vi "ReadSamples.vi"(8 "error in (no error)":errorcluster, 9 "Max num samples to keep":u32, 10 "Num samples to read":u32, 11 "FpgaRef5782 in":refnum<class "FpgaRef5782.lvclass">) -> (0 "error out":errorcluster, 2 "Data":dbl[][](array[numeric]), 3 "FpgaRef5782 out":refnum<class "FpgaRef5782.lvclass">)   [LabVIEW 2018, in "FpgaRef5782.lvclass"]
uses:
  FpgaRef5782.lvclass
  FpgaRef5782.lvclass/FpgaRef5782.ctl
  <vilib>/Utility/error.llb/Error Cluster From Error Code.vi
  <vilib>/rvi/errors/niLvFpgaAdjustHostInterfaceError.vi
  <vilib>/rvi/interface/nirviMethod/nirviMethod.xnode
  5782 FPGA ref.ctl
  <vilib>/FPGAPlugInAG/Dynamic/niLvFpga_ReadFifo_Dynamic.vi
  <vilib>/rvi/errors/niLvFpgaMergeErrorWithErrorCode.vi
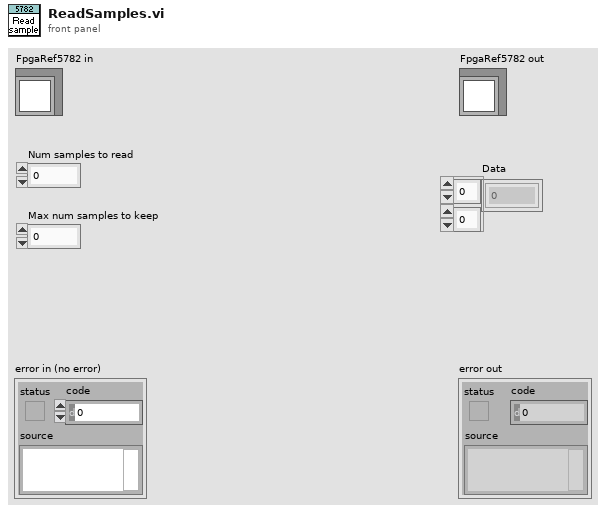
[diagram p1: front panel]
types:
  T1 = typedef "5782 FPGA ref.ctl" = refnum<k20>
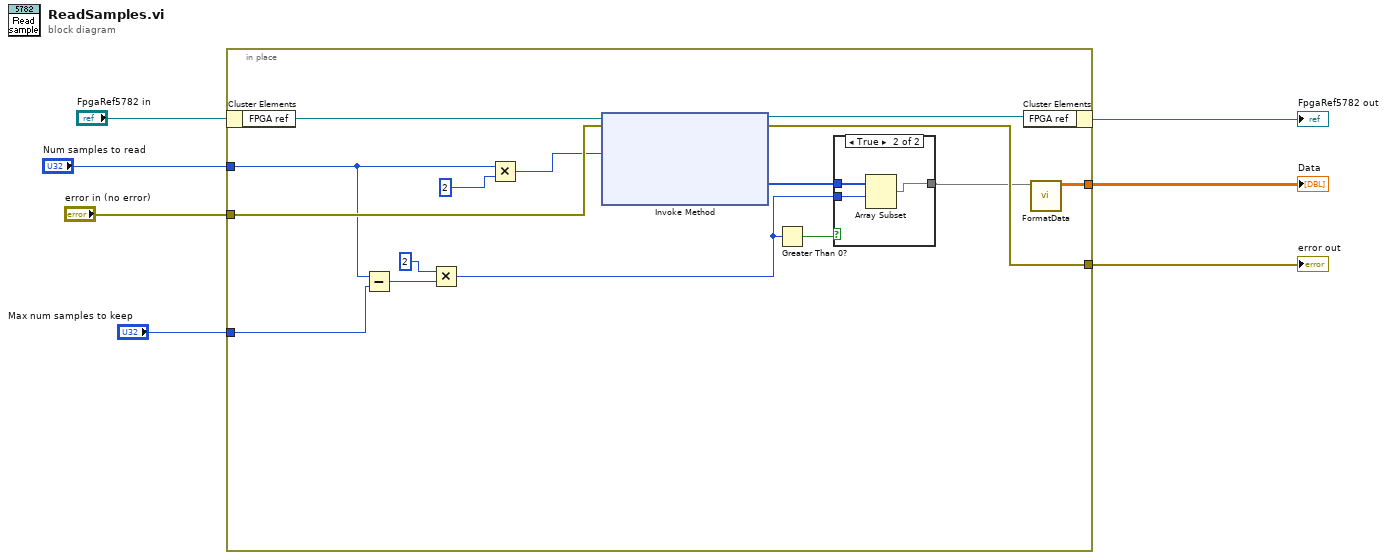
[diagram p0: block diagram]
diagram:
  n1 = in-place {
    in-place-border: [w21] -> w5
    in-place-border: [w20] -> w2
    in-place-border: "Num samples to read" -> [w9]
    in-place-border: "error in (no error)" -> [w18]
    in-place-border: "Max num samples to keep" -> [w10]
    n2 = in-place-cluster #1("FpgaRef5782 in") -> ("FPGA ref"=w19:T1)
    n3 = Subtract(x=w9, y=w10) -> (x-y=w15:u32)
    n4 = Multiply(x=u32 2, y=w15) -> (x*y=w14:u32)
    n5 = Multiply(x=w9, y=u32 2 ("x")) -> (x*y=w16:u32)
    n6 = xnode "Invoke Method"("FPGA VI Reference In"=w19, "error in"=w18, "Number of Elements"=w16) -> ("FPGA VI Reference Out"=w22:T1, "error out"=w20:errorcluster, "Data"=w12:u64[])  [unwired: 1 in, 1 out]
    n7 = Greater Than 0?(x=w14) -> (x > 0?=w8:bool)
    n8 = case shown="True" w8 {
      tunnel: w12 -> [w23 w26]
      tunnel: w14 -> [_ w25]
      tunnel: [w23 w24] -> w11
      frame False {
      }
      frame True {
        n9 = Array Subset(array=w26, index=w25) -> (w24:u64[])  [unwired: 1 in]
      }
    }
    n10 = in-place-cluster #1("FPGA ref"=w22) -> (→"FpgaRef5782 out":refnum<class "FpgaRef5782.lvclass">)
    n11 = call "FormatData.vi"("Raw data"=w11) -> ("Scaled"=w21:dbl[][])  [unwired: 10 in]
  }
  "error out" <- w2
  "Data" <- w5
